vi "3_ВПВычислениеСреднегоАрифметического.vi"() -> ()   [LabVIEW 2016]
panel:
  out "Average":dbl
  in  "Numeric 3":dbl
  in  "Numeric 2":dbl
  in  "Numeric":dbl
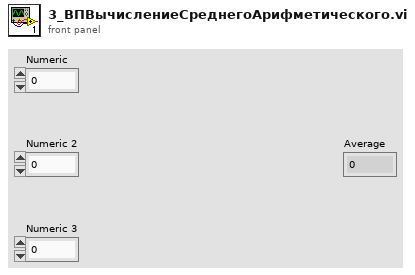
[diagram p1: front panel]
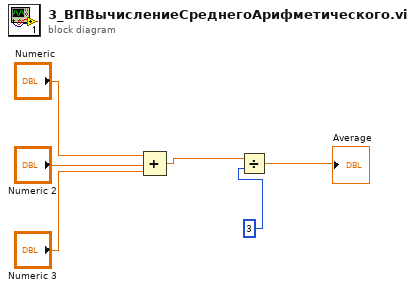
[diagram p0: block diagram]
diagram:
  n1 = Compound Arithmetic op=ADD("Numeric", "Numeric 2", "Numeric 3") -> (w4:dbl)
  n2 = Divide(x=w4, y=3) -> (x/y=→"Average":dbl)
